vi "Position to Direction.vi"(8 "Column":i32, 11 "Row":i32) -> (1 "Direction":T1)   [LabVIEW 2020, in "Bubble.lvclass"]
uses:
  Bubble.lvclass
  Type Defs/Direction Enum.ctl
  Type Defs/SB Type Defs.lvlib
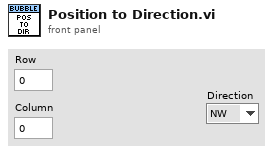
[diagram p1: front panel]
types:
  T1 = typedef "SB Type Defs.lvlib/Direction Enum.ctl" = enum16{"NW", "N", "NE", "E", "SE", "S", "SW", "W"}
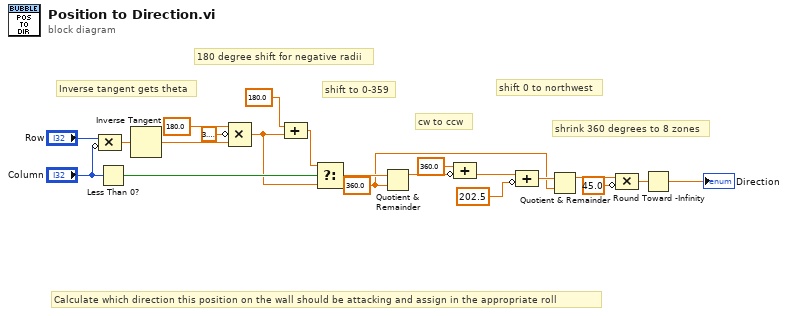
[diagram p0: block diagram]
diagram:
  w12 = 360.0 ("y")
  # "cw to ccw"
  # "shrink 360 degrees to 8 zones"
  # "shift 0 to northwest"
  # "shift to 0-359"
  # "180 degree shift for negative radii"
  # "Inverse tangent gets theta"
  # "Calculate which direction this position on the wall should be attacking and assign in the appropriate roll"
  n1 = Less Than 0?(x="Column") -> (x < 0?=w18:bool)
  n2 = Compound Arithmetic op=MULTIPLY("Row", invert "Column") -> (w20:dbl)
  n3 = Inverse Tangent(1:w20) -> (0:w7:dbl)
  n4 = Compound Arithmetic op=MULTIPLY(180.0 ("value"), invert 3.141592653589793, w7) -> (w5:dbl)
  n5 = Compound Arithmetic op=ADD(180.0 ("value"), w5) -> (w17:dbl)
  n6 = Select(t=w17, s=w18, f=w5) -> (s? t:f=w15:dbl)
  n7 = Quotient & Remainder(x=w15, y=w12) -> (x-y*floor(x/y)=w3:dbl)  [unwired: 1 out]
  n8 = Compound Arithmetic op=ADD(360.0 ("value"), invert w3) -> (w1:dbl)
  n9 = Compound Arithmetic op=ADD(w1, invert 202.5 ("value")) -> (w13:dbl)
  n10 = Quotient & Remainder(x=w13, y=w12) -> (x-y*floor(x/y)=w11:dbl)  [unwired: 1 out]
  n11 = Compound Arithmetic op=MULTIPLY(w11, invert 45.0 ("value")) -> (w9:dbl)
  n12 = Round Toward -Infinity(1:w9) -> (0:→"Direction":dbl)
